vi "Write Channels Names.vi"(8 "error in (no error)":errorcluster, 10 "Channels Names":string[](array[string]), 11 "Data List in":refnum<class "Data List.lvclass">) -> (0 "error out":errorcluster, 3 "Data List out":refnum<class "Data List.lvclass">)   [LabVIEW 2020, in "Data List.lvclass"]
uses:
  Data List.lvclass
  Data List.lvclass/Data List.ctl
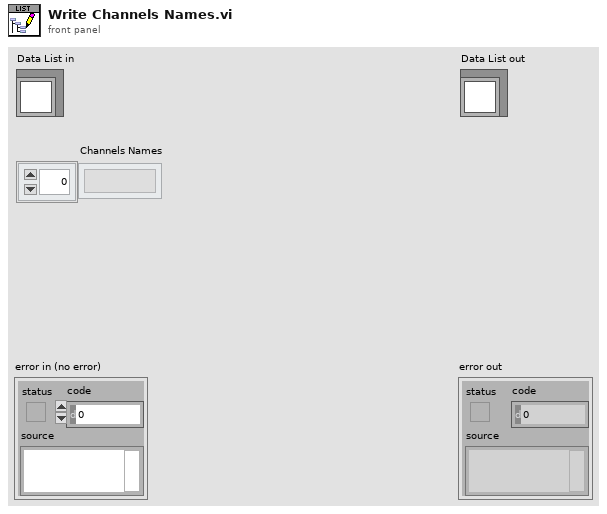
[diagram p1: front panel]
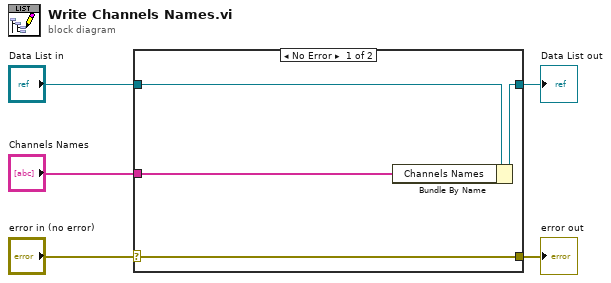
[diagram p0: block diagram]
diagram:
  n1 = case shown="No Error" "error in (no error)" {
    selector: "error in (no error)" -> [w9 w10]
    tunnel: [w9 w10] -> w4
    tunnel: [w7 w11] -> w2
    tunnel: "Data List in" -> [w8 w11]
    tunnel: "Channels Names" -> [w6 _]
    frame No Error {
      n2 = Bundle By Name(cluster=w8, "Channels Names"=w6) -> (w7:refnum<class "Data List.lvclass">)
    }
    frame Error {
    }
  }
  "error out" <- w4
  "Data List out" <- w2
